vi "ImageType.vi"(0 "ImageType":string) -> (1 "TypeName":string, 2 "ShutterState":bool, 3 "Comparison?":bool, 4 "Error":bool)   [LabVIEW 2014]
uses:
  globals/AzCamGlobals.vi
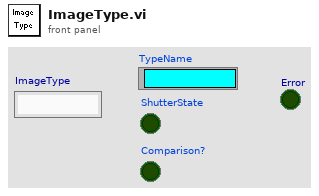
[diagram p1: front panel]
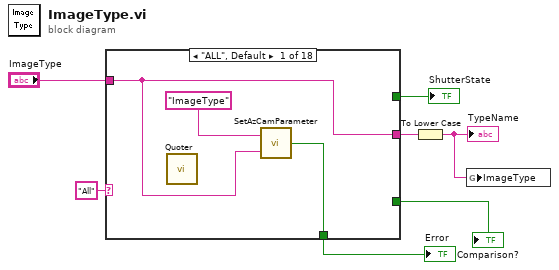
[diagram p0: block diagram]
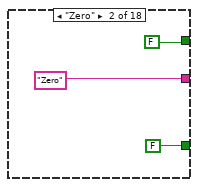
[diagram p2: hidden frame]
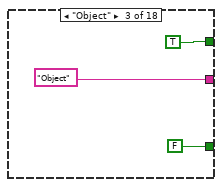
[diagram p3: hidden frame]
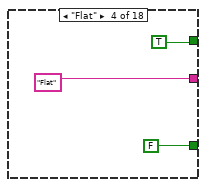
[diagram p4: hidden frame]
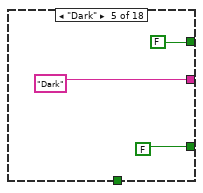
[diagram p5: hidden frame]
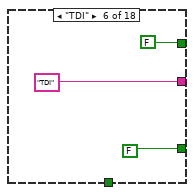
[diagram p6: hidden frame]
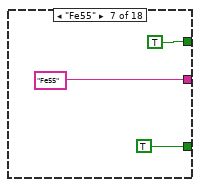
[diagram p7: hidden frame]
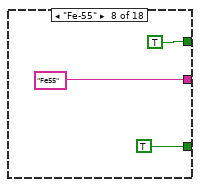
[diagram p8: hidden frame]
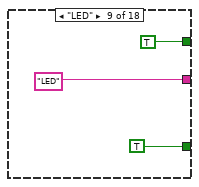
[diagram p9: hidden frame]
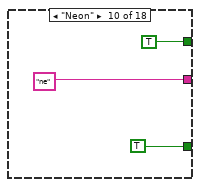
[diagram p10: hidden frame]
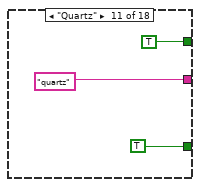
[diagram p11: hidden frame]
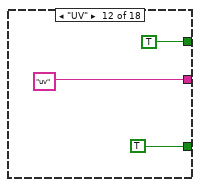
[diagram p12: hidden frame]
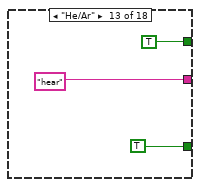
[diagram p13: hidden frame]
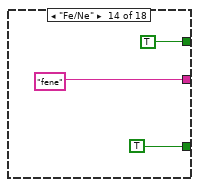
[diagram p14: hidden frame]
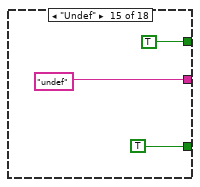
[diagram p15: hidden frame]
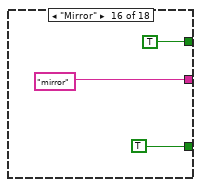
[diagram p16: hidden frame]
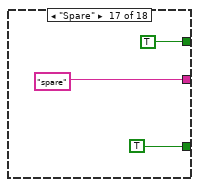
[diagram p17: hidden frame]
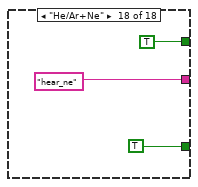
[diagram p18: hidden frame]
diagram:
  n1 = case shown="\"ALL\", Default" "All" {
    tunnel: [_ FALSE ("ShutterCase") TRUE ("ShutterCase") TRUE ("ShutterCase") FALSE ("ShutterCase") FALSE ("ShutterCase") TRUE ("ShutterCase") TRUE ("ShutterCase") TRUE ("ShutterCase") TRUE ("ShutterCase") TRUE ("ShutterCase") TRUE ("ShutterCase") TRUE ("ShutterCase") TRUE ("ShutterCase") TRUE ("ShutterCase") TRUE ("ShutterCase") TRUE ("ShutterCase") TRUE ("ShutterCase")] -> w6
    tunnel: [w8 "Zero" "Object" "Flat" "Dark" "TDI" "Fe55" "Fe55" "LED" "ne" "quartz" "uv" "hear" "fene" "undef" "mirror" "spare" "hear_ne"] -> w7
    tunnel: [_ FALSE ("ShutterCase") FALSE ("ShutterCase") FALSE ("ShutterCase") FALSE ("ShutterCase") FALSE ("ShutterCase") TRUE ("ShutterCase") TRUE ("ShutterCase") TRUE ("ShutterCase") TRUE ("ShutterCase") TRUE ("ShutterCase") TRUE ("ShutterCase") TRUE ("ShutterCase") TRUE ("ShutterCase") TRUE ("ShutterCase") TRUE ("ShutterCase") TRUE ("ShutterCase") TRUE ("ShutterCase")] -> w5
    tunnel: "ImageType" -> [w8 _ _ _ _ _ _ _ _ _ _ _ _ _ _ _ _ _]
    tunnel: [w9 _ _ _ _ _ _ _ _ _ _ _ _ _ _ _ _ _] -> w1
    frame "ALL", Default {
      n2 = call "Quoter.vi"() -> ()  [unwired: 1 in, 1 out]
      n3 = call "SetAzCamParameter.vi"("Value"=w8, "Parameter"="ImageType") -> ("Error"=w9:bool)
    }
    frame "Zero" {
    }
    frame "Object" {
    }
    frame "Flat" {
    }
    frame "Dark" {
    }
    frame "TDI" {
    }
    frame "Fe55" {
    }
    frame "Fe-55" {
    }
    frame "LED" {
    }
    frame "Neon" {
    }
    frame "Quartz" {
    }
    frame "UV" {
    }
    frame "He/Ar" {
    }
    frame "Fe/Ne" {
    }
    frame "Undef" {
    }
    frame "Mirror" {
    }
    frame "Spare" {
    }
    frame "He/Ar+Ne" {
    }
  }
  "ShutterState" <- w6
  "Comparison?" <- w5
  "Error" <- w1
  n4 = To Lower Case(string=w7) -> (all lower case string=w4:string)
  "TypeName" <- w4
  n5 = global write "AzCamGlobals.vi" "ImageType"(w4) -> ()
